vi "DataTypeTest.vi"() -> ()   [LabVIEW 2014]
uses:
  Packages/CSPP_Core/Libraries/Utilities/CS++Utilities.lvlib
panel:
  out "Error Out":errorcluster
  out "TypeDescriptor":string
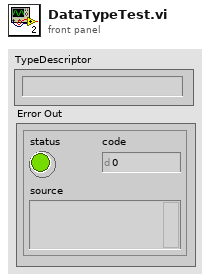
[diagram p1: front panel]
types:
  T1 = cluster{"channel name (\"CHANNEL1\")":string, "probe attenuation (1:1.0)":dbl, "vertical range (10.0 V)":dbl[unit], "vertical offset (0.0 V)":dbl[unit], "channel enabled (True)":bool, "vertical coupling (DC)":i32}
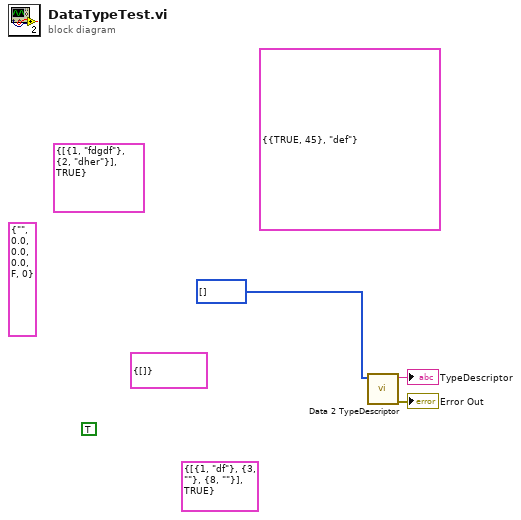
[diagram p0: block diagram]
diagram:
  (unwired) TRUE
  (unwired) T1 {"channel name (\"CHANNEL1\")"="", "probe attenuation (1:1.0)"=0.0, "vertical range (10.0 V)"=0.0, "vertical offset (0.0 V)"=0.0, "channel enabled (True)"=FALSE, "vertical coupling (DC)"=0} ("output cluster")
  (unwired) cluster{cluster{bool, i32}, string} {{TRUE, 45}, "def"}
  (unwired) cluster{cluster{i32, string}[], bool} {[{1, "fdgdf"}, {2, "dher"}], TRUE}
  (unwired) cluster{cluster{i32, string}[], bool} {[{1, "df"}, {3, ""}, {8, ""}], TRUE}
  (unwired) cluster{cluster{i32, string}[]} {[]}
  n1 = call "Data 2 TypeDescriptor.vi"("Data"=i32[] []) -> ("Error Out"=→"Error Out":errorcluster, "TypeDescriptor"=→"TypeDescriptor":string)  [unwired: 9 in]
